vi "Get Log File Specification.vi"(8 "error in (no error)":errorcluster, 10 "Log File Specification type":refnum<class "Log File Specification.lvclass">, 11 "Segmented Log in":refnum<class "Segmented Log.lvclass">) -> (0 "error out":errorcluster, 1 "Is expected type?":bool, 2 "Log File Specification":refnum<class "Log File Specification.lvclass">, 3 "Segmented Log out":refnum<class "Segmented Log.lvclass">)   [LabVIEW 2015, in "Segmented Log.lvclass"]
uses:
  Segmented Log.lvclass
  Log File Specifications/Log File Specification/Log File Specification.lvclass
  Segmented Log.lvclass/Segmented Log.ctl
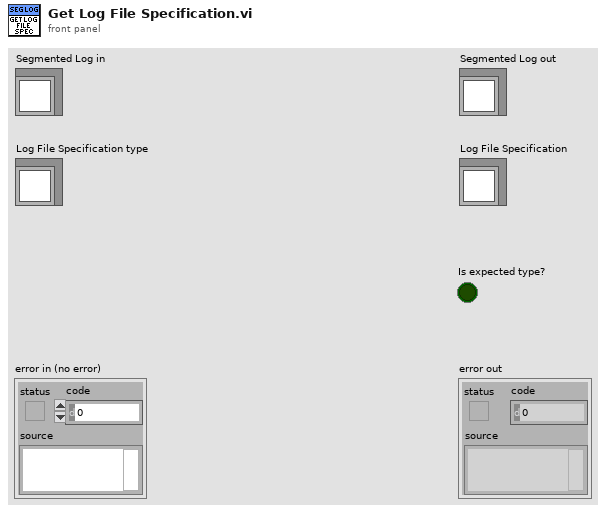
[diagram p1: front panel]
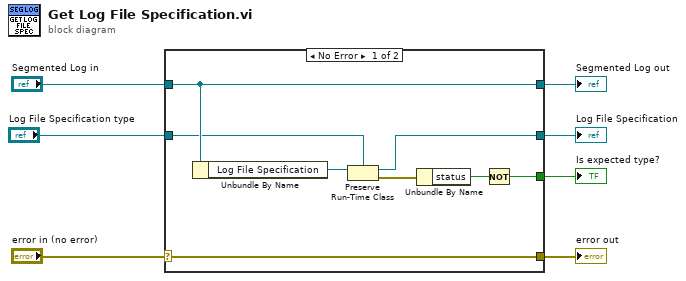
[diagram p0: block diagram]
diagram:
  n1 = case shown="No Error" "error in (no error)" {
    selector: "error in (no error)" -> [w15 w17]
    tunnel: [w15 w17] -> w6
    tunnel: [w14 w18] -> w4
    tunnel: "Segmented Log in" -> [w14 w18]
    tunnel: [w11 w16] -> w3
    tunnel: "Log File Specification type" -> [w12 w16]
    tunnel: [w8 _] -> w1
    frame No Error {
      n2 = Unbundle By Name(w14) -> ("Log File Specification"=w13:refnum<class "Log File Specification.lvclass">)
      n3 = Preserve Run-Time Class(object in=w13, 2:w12) -> (object out=w11:refnum<class "Log File Specification.lvclass">, error out=w10:errorcluster)  [unwired: 1 in]
      n4 = Unbundle By Name(w10) -> ("status"=w9:bool)
      n5 = Not(x=w9) -> (.not. x?=w8:bool)
    }
    frame Error {
    }
  }
  "error out" <- w6
  "Segmented Log out" <- w4
  "Log File Specification" <- w3
  "Is expected type?" <- w1
